vi "Get Supported Targets.vi"(8 "error in":errorcluster, 11 "JSON_RPC_Interface configuration in":refnum<class "JSON_RPC_Interface configuration.lvclass">) -> (0 "error out":errorcluster, 2 "supported targets":T1[](array[typedef]), 3 "JSON_RPC_Interface configuration out":refnum<class "JSON_RPC_Interface configuration.lvclass">)   [LabVIEW 2018, in "JSON_RPC_Interface configuration.lvclass"]
doc: "Provides an interface for determining the targets supported by a given module configuration/runtime class pairing. This should be overridden by any useful child class."
uses:
  JSON_RPC_Interface configuration.lvclass
  <vilib>/NI/Tag Bus Module Framework/root configuration/Target Types.ctl
  <vilib>/NI/Tag Bus Module Framework/root configuration/TBM configuration.lvclass
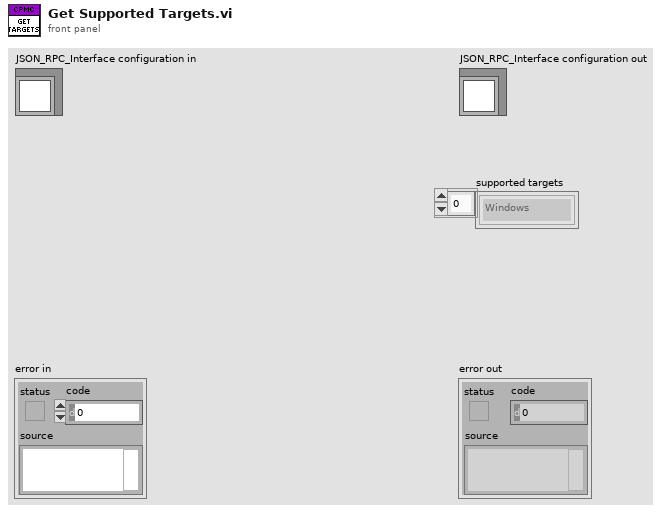
[diagram p1: front panel]
types:
  T1 = typedef "TBM configuration.lvclass/Target Types.ctl" = enum16{"Windows", "Mac", "Linux", "Linux RT ARM", "VxWorks", "Pharlap", "Other", "Linux RT x64"}
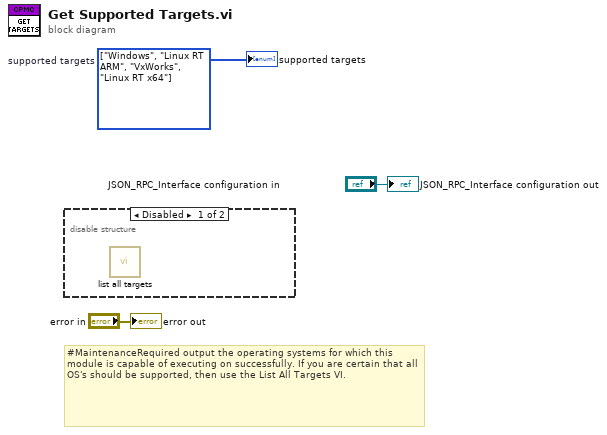
[diagram p0: block diagram]
diagram:
  w1 = T1[] [enum."Windows", enum."Linux RT ARM", enum."VxWorks", enum."Linux RT x64"] items=["Windows", "Mac", "Linux", "Linux RT ARM", "VxWorks", "Pharlap", "Other", "Linux RT x64"]  # supported targets
  # "#MaintenanceRequired output the operating systems for which this module is capable of executing on successfully. If you are certain that all OS's should be supported, then use the List All Targets VI."
  n1 = disable-structure shown="Disabled" {
    frame Disabled {
      n2 = call <vilib>:"list all targets.vi"() -> ()  [unwired: 11 in, 1 out]
    }
    frame Enabled {
    }
  }
  "error out" <- "error in"
  "JSON_RPC_Interface configuration out" <- "JSON_RPC_Interface configuration in"
  "supported targets" <- w1
